vi "chart get x axis.vi"(8 "error in (no error)":errorcluster, 11 "chart":u32) -> (0 "error out":errorcluster, 3 "function return":u32)   [LabVIEW 2015, in "xlsxwriter.lvlib"]
doc: "lxw_chart_axis chart_get_x_axis(lxw_chart chart);"
uses:
  xlsxwriter.lvlib
  xlsxwriter.dll
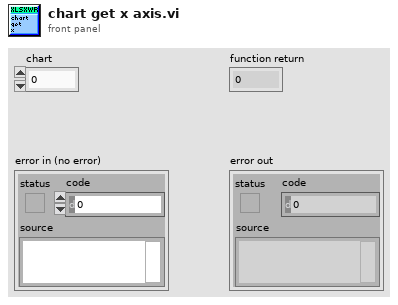
[diagram p1: front panel]
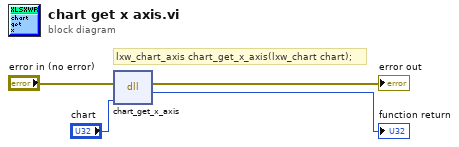
[diagram p0: block diagram]
diagram:
  # "lxw_chart_axis chart_get_x_axis(lxw_chart chart);"
  n1 = dll-call lib="C:/Users/WDAGUtilityAccount/Desktop/lv_vis_added_cell/xlsxwriter.*" fn="chart_get_x_axis"(error in="error in (no error)", "chart"="chart") -> (error out=→"error out":errorcluster, →"function return":u32)  [unwired: 3 in, 1 out]
